vi "Edgertronic Main.vi"() -> ()   [LabVIEW 2015]
panel:
  out "Settings":string
  in  "URL":string="192.168.1.123"
  in  "Exposure (1/sec)":i32(knob)=10 min=10 max=250000 step=1 scale=10.0..250000.0
  out "Pretrigger Fill Level":cluster{u8, u8, u8}(slide)={100, 46, 32} scale=0.0..100.0
  in  "Tab Control":T1(tab)=enum."Parameters"
  in  "Configure Camera:":T2={"Duration (sec)"=1.0, "Subsample?"=FALSE, "Force Mono?"=FALSE, "Pretrigger (%)"=50.0, "ISO"=500.0, "Horizontal"=873.0, "Vertical"=630.0, "Frame Rate (fps)"=1000.0, "Genlock"=enum."Off", "Overclock"=enum."Off", "Exposure (1/sec)"=1500.0, "MultiShot"=1} {"Exposure (1/sec)" min=4e-06 max=250000.0 step=1.0 scale=10.0..250000.0; "Frame Rate (fps)" min=0.1 max=25000.0 step=1.0 scale=0.1..25000.0; "Vertical" min=192.0 max=1280.0 step=1.0 scale=96.0..1024.0; "Horizontal" min=192.0 max=1280.0 step=1.0 scale=192.0..1280.0; "ISO" min=0.0 max=1600.0 step=1.0 scale=400.0..1600.0; "Pretrigger (%)" min=0.0 max=100.0 step=1.0 scale=0.0..100.0; "Duration (sec)" min=0.0}
  in  "Run":bool
  out "Cam Status":T3={"Pretrigger Fill Level"=100, "IS Temp"=30.0, "State"=6, "dacvrefadc"="187", "Flags"={"Storage full"=FALSE, "Storage missing"=FALSE, "USB Storage installed"=FALSE, "SD Card installed"=TRUE, "USB full"=FALSE, "SD Card full"=FALSE, "Bad storage"=FALSE, "Net Configured"=FALSE, "Net unmountable"=FALSE, "Net full"=FALSE, "Storage full 11"=FALSE, "Storage full 12"=FALSE, "Storage full 13"=FALSE, "Storage full 14"=FALSE, "Storage full 15"=FALSE, "Storage full 16"=FALSE, "Storage full 17"=FALSE, "Genlock - no signal"=FALSE, "Genlock - config err"=FALSE}, "FPGA Temp"=34.0, "Camera time"=timestamp(1465914006 s since 1904-01-01)} {"Camera time" format="%<%X>T"; "FPGA Temp" scale=10.0..50.0; "State" items=["Unconfigured", "Calibrating", "Running", "Triggered", "Saving", "Pretrigger full", "Trigger Canceled", "Save Canceled"]; "IS Temp" scale=10.0..50.0; "Pretrigger Fill Level" scale=0.0..100.0}
  out "Cam Info":T4={"Hardware Build Date"=timestamp(3503952000 s since 1904-01-01), "Software Build Date"=timestamp(3493324800 s since 1904-01-01), "FPGA Initialized"="1", "Hardware Revision"="6", "Model"="1", "Home Dir"="/home/root/ss-web", "IR Filter"="1", "Mac Address"="00:1B:C5:09:61:4D", "Serial Console Enabled"="false", "Serial number"="333", "FPGA Version"="70", "Hardware Configuration"="1", "Connection Information:"="HTTP/1.0 200 OK\r\nContent-Type: text/html; charset=utf-8\r\nContent-Length: 313\r\nConnection: close\r\nDate: Tue, 14 Jun 2016 14:20:06 GMT\r\nServer: lighttpd/1.4.11 (edgertonic slow motion camera)"} {"Software Build Date" format="%<%x>T"; "Hardware Build Date" format="%<%x>T"}
  in  "Download":bool
  out "Last movie":string
  in  "Movies":i32(listbox)
  in  "Controls":T5
  out "Storage Status":cluster{"Storage Status":u8, "String":string}={"Storage Status"=57, "String"="2.0GB  used of 7.9GB"} {"Storage Status" scale=0.0..100.0}
  in  "Stop Button":bool
  in  "Zoom Factor":sgl(slide)=0.5 scale=0.0..1.0
  out "Image":picture
  # "Sun Jun 26 20:30 2016\t\n\nSensitivity:\t400\tISO\n\nShutter:\t1/500\tSeconds\n\nFrame Rate:\t498.256\tfps\n\nHorizontal:\t1264\tPixels\nVertical:\t1008\tPixels"
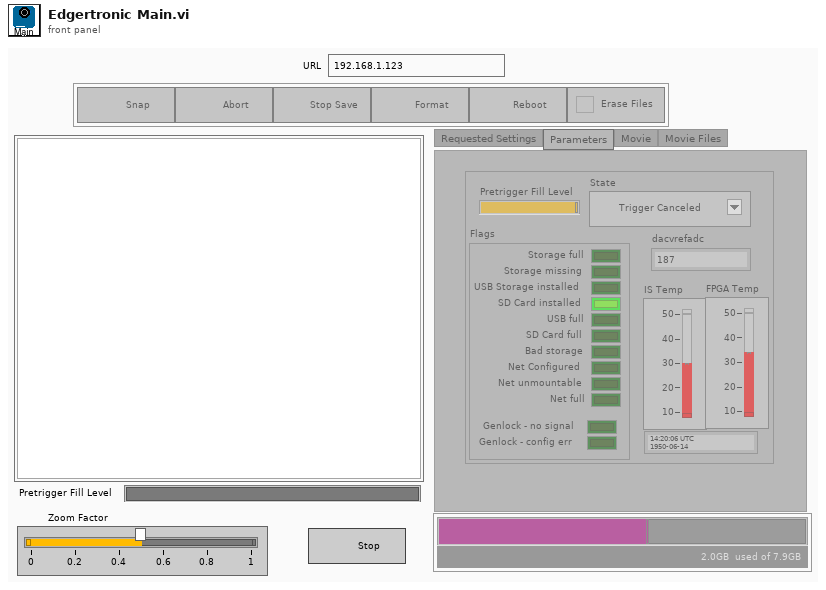
[diagram p1: front panel]
types:
  T1 = enum32{"Requested Settings", "Parameters", "Movie", "Movie Files"}
  T2 = cluster{"Duration (sec)":dbl, "Subsample?":bool, "Force Mono?":bool, "Pretrigger (%)":dbl, "ISO":dbl, "Horizontal":dbl, "Vertical":dbl, "Frame Rate (fps)":dbl, "Genlock":enum16{"Off", "Master", "Slave"}, "Overclock":enum16{"Off", "A level", "B Level", "C Level", "D Level"}, "Exposure (1/sec)":dbl, "MultiShot":i16}
  T3 = cluster{"Pretrigger Fill Level":u8, "IS Temp":dbl, "State":u16, "dacvrefadc":string, "Flags":cluster{"Storage full":bool, "Storage missing":bool, "USB Storage installed":bool, "SD Card installed":bool, "USB full":bool, "SD Card full":bool, "Bad storage":bool, "Net Configured":bool, "Net unmountable":bool, "Net full":bool, "Storage full 11":bool, "Storage full 12":bool, "Storage full 13":bool, "Storage full 14":bool, "Storage full 15":bool, "Storage full 16":bool, "Storage full 17":bool, "Genlock - no signal":bool, "Genlock - config err":bool}, "FPGA Temp":dbl, "Camera time":timestamp}
  T4 = cluster{"Hardware Build Date":timestamp, "Software Build Date":timestamp, "FPGA Initialized":string, "Hardware Revision":string, "Model":string, "Home Dir":string, "IR Filter":string, "Mac Address":string, "Serial Console Enabled":string, "Serial number":string, "FPGA Version":string, "Hardware Configuration":string, "Connection Information:":string}
  T5 = cluster{"Trigger":bool, "Cancel":bool, "Stop Save":bool, "Format":bool, "Reboot":bool, "Trash":bool}
  T6 = enum8{"Enabled", "Disabled", "Disabled and Grayed Out"}
  T7 = cluster{"Build Date":timestamp, "Software Build Date":timestamp, "FPGA Initialized":string, "Hardware Revision":string, "Model Number":string, "Home Dir":string, "IR Filter":string, "Mac Address":string, "Serial Console Enabled":string, "Serial number":string, "FPGA Version":string, "Hardware Configuration":string, "Connection Information:":string}
  T8 = cluster{"Connection Information:":string, "Last Saved File Name":string}
  T9 = cluster{"Requested Genlock":string, "Duration ":string, "Overclock ":string, "Requested Horizontal ":string, "Requested Pretrigger ":string, "Requested Duration ":string, "Vertical ":string, "Requested Vertical ":string, "Reqested Frame Rate ":string, "Frame Rate ":string, "Horizontal ":string, "Exposure ":string, "Genlock ":string, "Subsample ":string, "Requested Exposure ":string, "Iso ":string, "Requested Overclock":string, "Requested Subsample":string, "Pretrigger":string, "Requested Iso":string, "Multishot":string, "Gain":string}
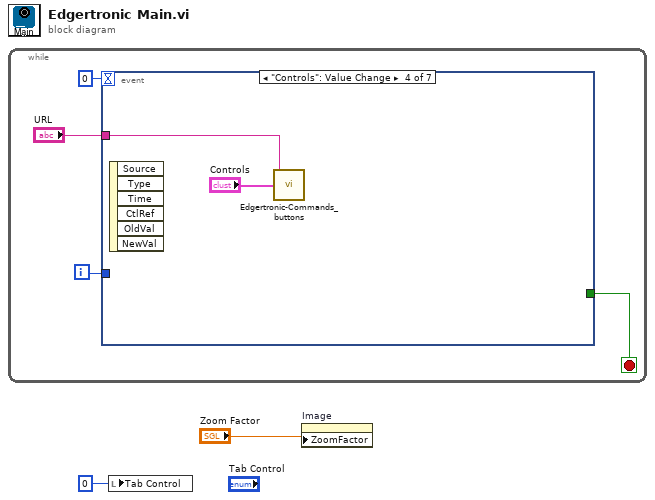
[diagram p0: block diagram]
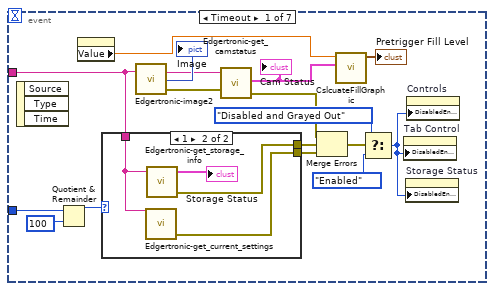
[diagram p2: hidden frame]
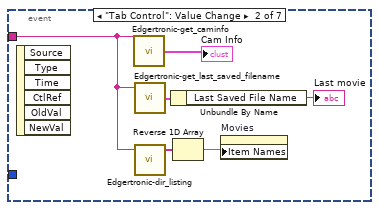
[diagram p4: hidden frame]
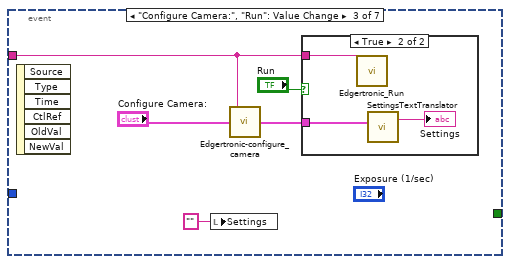
[diagram p5: hidden frame]
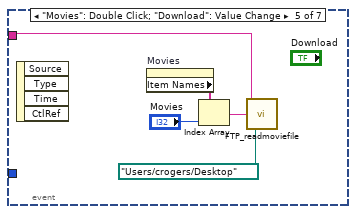
[diagram p7: hidden frame]
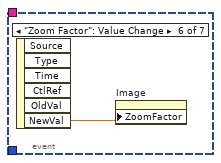
[diagram p8: hidden frame]
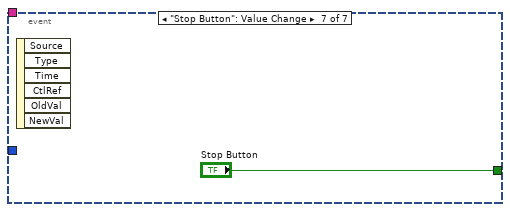
[diagram p9: hidden frame]
diagram:
  n1 = while {
    i -> [w4]
    stop <- w5 stop-if-true
    n2 = event shown="[3] \"Controls\": Value Change" {
      selector: _ -> [_ _ _ _ _ _ _]
      dyn-events: _ -> [_ _ _ _ _ _ _]
      timeout: 0 -> [_ _ _ _ _ _ _]
      tunnel: [_ _ _ _ _ _ "Stop Button"] -> w5
      tunnel: "URL" -> [w10 w30 w34 w42 w45 _ _]
      tunnel: w4 -> [w21 _ _ _ _ _ _]
      event Timeout {
        n3 = event-data() -> ()  [unwired: 1 in, 3 out]
        n4 = Quotient & Remainder(x=w21, y=100) -> (x-y*floor(x/y)=w19:i32)  [unwired: 1 out]
        n5 = property class="DigNum (strict)"() -> ("Value"=w7:dbl)  [unwired: 2 in, 2 out]
        n6 = case shown="1" w19 {
          tunnel: w10 -> [_ w26]
          tunnel: [_ w24] -> w18
          tunnel: [_ w23] -> w17
          frame 0, Default {
          }
          frame 1 {
            n7 = call "Edgertronic-get_current_settings.vi"("URL"=w26) -> ("error out"=w23:errorcluster)  [unwired: 3 in, 1 out]
            n8 = call "Edgertronic-get_storage_info.vi"("URL"=w26) -> ("error out"=w24:errorcluster, "Storage Status"=→"Storage Status":cluster{"Storage Status":u8, "String":string})  [unwired: 2 in, 1 out]
          }
        }
        n9 = call "Edgertronic-image2.vi"("URL"=w10) -> ("error out"=w12:errorcluster, "new picture"=→"Image":picture)  [unwired: 2 in, 1 out]
        n10 = call "Edgertronic-get_camstatus.vi"("error in (no error)"=w12, "URL"=w10) -> ("error out"=w11:errorcluster, "Status"=w9:T3)  [unwired: 1 in, 1 out]
        "Cam Status" <- w9
        n11 = Merge Errors(w11, w18, w17) -> (w16:errorcluster)
        n12 = call "CslcuateFillGraphic.vi"("Status"=w9, "% trigger"=w7) -> ("Pretrigger Fill Level"=→"Pretrigger Fill Level":cluster{u8, u8, u8})  [unwired: 9 in]
        n13 = Select(t=T6."Disabled and Grayed Out" ("Disabled"), s=w16, f=T6."Enabled" ("Disabled")) -> (s? t:f=w13:T6)
        n14 = property on="Tab Control" class="TabCtl (strict)"("DisabledEnum"=w13) -> ()  [unwired: 2 in, 2 out]
        n15 = property on="Storage Status" class="Clust (strict)"("DisabledEnum"=w13) -> ()  [unwired: 2 in, 2 out]
        n16 = property on="Controls" class="Clust"("DisabledEnum"=w13) -> ()  [unwired: 2 in, 2 out]
      }
      event "Tab Control": Value Change {
        n17 = event-data() -> ()  [unwired: 1 in, 6 out]
        n18 = call "Edgertronic-get_caminfo.vi"("URL"=w30) -> ("Cam Info"=→"Cam Info":T7)  [unwired: 3 in, 1 out]
        n19 = call "Edgertronic-get_last_saved_filename.vi"("URL"=w30) -> ("Last Saved File Name:"=w29:T8)  [unwired: 3 in, 1 out]
        n20 = call "Edgertronic-dir_listing.vi"("URL"=w30) -> ("Movies"=w31:string[])  [unwired: 2 in, 2 out]
        n21 = Unbundle By Name(w29) -> ("Last Saved File Name"=→"Last movie":string)
        n22 = Reverse 1D Array(array=w31) -> (reversed array=w27:string[])
        n23 = property on="Movies" class="LstBox (strict)"("Item Names"=w27) -> ()  [unwired: 2 in, 2 out]
      }
      event "Configure Camera:", "Run": Value Change {
        n24 = event-data() -> ()  [unwired: 1 in, 6 out]
        n25 = local write "Settings"("" ("Settings")) -> ()
        n26 = call "Edgertronic-configure_camera.vi"("Configure Camera:"="Configure Camera:", "URL"=w34) -> ("Current Settings:"=w35:T9)  [unwired: 2 in, 1 out]
        n27 = case shown="True" "Run" {
          tunnel: w35 -> [_ w39]
          tunnel: w34 -> [_ w38]
          frame False {
          }
          frame True {
            n28 = call "Edgertronic_Run.vi"("URL"=w38) -> ()  [unwired: 4 in, 1 out]
            n29 = call "SettingsTextTranslator.vi"("Current Settings:"=w39) -> ("Settings"=→"Settings":string)  [unwired: 2 in]
          }
        }
      }
      event "Controls": Value Change {
        n30 = event-data() -> ()  [unwired: 1 in, 6 out]
        n31 = call "Edgertronic-Commands_buttons.vi"("Controls"="Controls", "URL"=w42) -> ()  [unwired: 2 in, 2 out]
      }
      event "Movies": Double Click; "Download": Value Change {
        n32 = event-data() -> ()  [unwired: 1 in, 4 out]
        n33 = property on="Movies" class="LstBox (strict)"() -> ("Item Names"=w47:string[])  [unwired: 2 in, 2 out]
        n34 = Index Array(array=w47, index="Movies") -> (element=w44:string)
        n35 = call "FTP_readmoviefile.vi"("local path"=path "/Users/crogers/Desktop", "Movie name"=w44, "URL"=w45) -> ()  [unwired: 3 in]
      }
      event "Zoom Factor": Value Change {
        n36 = event-data() -> ("NewVal"=w48:sgl)  [unwired: 1 in, 5 out]
        n37 = property on="Image" class="Pict"("ZoomFactor"=w48) -> ()  [unwired: 2 in, 2 out]
      }
      event "Stop Button": Value Change {
        n38 = event-data() -> ()  [unwired: 1 in, 6 out]
      }
    }
  }
  n39 = local write "Tab Control"(0) -> ()
  n40 = property on="Image" class="Pict"("ZoomFactor"="Zoom Factor") -> ()  [unwired: 2 in, 2 out]
